vi "Replace String Value.vi"(0 "MICS Value In":string, 5 "Search":string, 7 "Replace By":string) -> (8 "MICS Value Out":string)   [LabVIEW 2010]
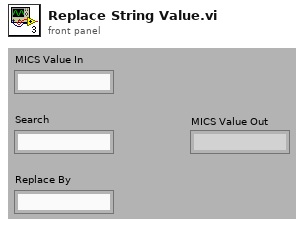
[diagram p1: front panel]
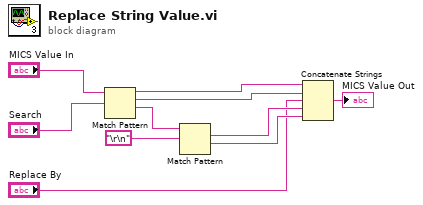
[diagram p0: block diagram]
diagram:
  n1 = Match Pattern(string="MICS Value In", regular expression="Search") -> (before substring=w7:string, match substring=w5:string, after substring=w9:string)  [unwired: 1 in, 1 out]
  n2 = Match Pattern(string=w9, regular expression="\r\n") -> (match substring=w4:string, after substring=w3:string)  [unwired: 1 in, 2 out]
  n3 = Concatenate Strings(w7, w5, "Replace By", w4, w3) -> (→"MICS Value Out":string)
